vi "Save_Position_Checking.vi"(2 "Traverse Name":string, 3 "Error String":string, 4 "Model       Roll      Pitch       Yaw (deg)":sgl[](array[numeric]) format="%#.2f", 5 "Position":sgl[](array[numeric])=[0.0, 200.0, 40.0] format="%.2f") -> ()   [LabVIEW 2018]
uses:
  Collision_Detection/Triangles/EnFlo specific/Collision Detection global.vi
  Globals/Constants_global.vi
  Globals/Trav_pos_global.vi
panel:
  out "appended array":string[](array[string])
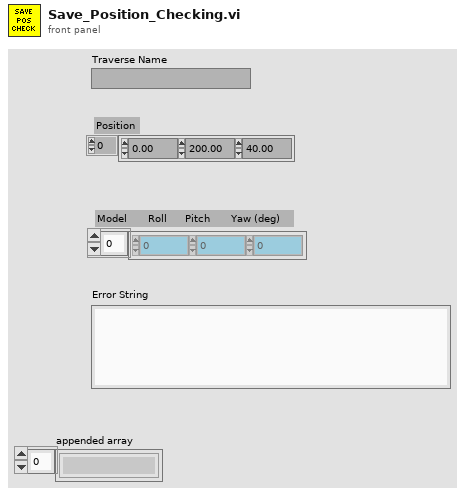
[diagram p1: front panel]
types:
  T1 = typedef "Traverse_cluster.ctl" = cluster{"Start X":sgl, "Start Y":sgl, "Start Z":sgl, "End X":sgl, "End Y":sgl, "End Z":sgl, "No. of pts.":i32, "Spacing":T2, "Filename":path, "Tunnel Speed":dbl, "Averaging time (min)":dbl, "Extra Commands":string, "Carrier_1 Q (l/min)":dbl, "Carrier_2 Q (l/min)":dbl, "Trace Gas Concentration (%)":dbl, "Specific Arguments":string, "Comments":string, "Row No":i32, "Row Type Selector":T3, "Completion time":string, "Row Duration (mins)":dbl, "No. of Valid pts.":i32, "Meas Setup File":string}
  T2 = typedef "Spacing.ctl" = enum16{"Linear", "Log", "Gauss", "Specified", "N/A"}
  T3 = typedef "Multi_run_mode.ctl" = enum16{"Move Traverse Only", "Set Tunnel Speed Only", "Set Source Only", "Set Measurement Conditions", "Single Measurement", "Vertical Profile", "Lateral Profile", "Longitudinal Profile", "Multi-Axis Profile", "Explore Volume", "Auto Calibrate", "Meas Fast FID Bkgnd", "Check Beam Power", "Scanning Valve Measurement", "Run VI Named:", "Set ADAM Ch", "Wait (minutes)", "Send Message", "Synchronize With:", "Fall Back to this Row", "Turn Off Row Repeating", "Traverse 3D Volume", "Blank Row", "Jump to Fall Back Row"}
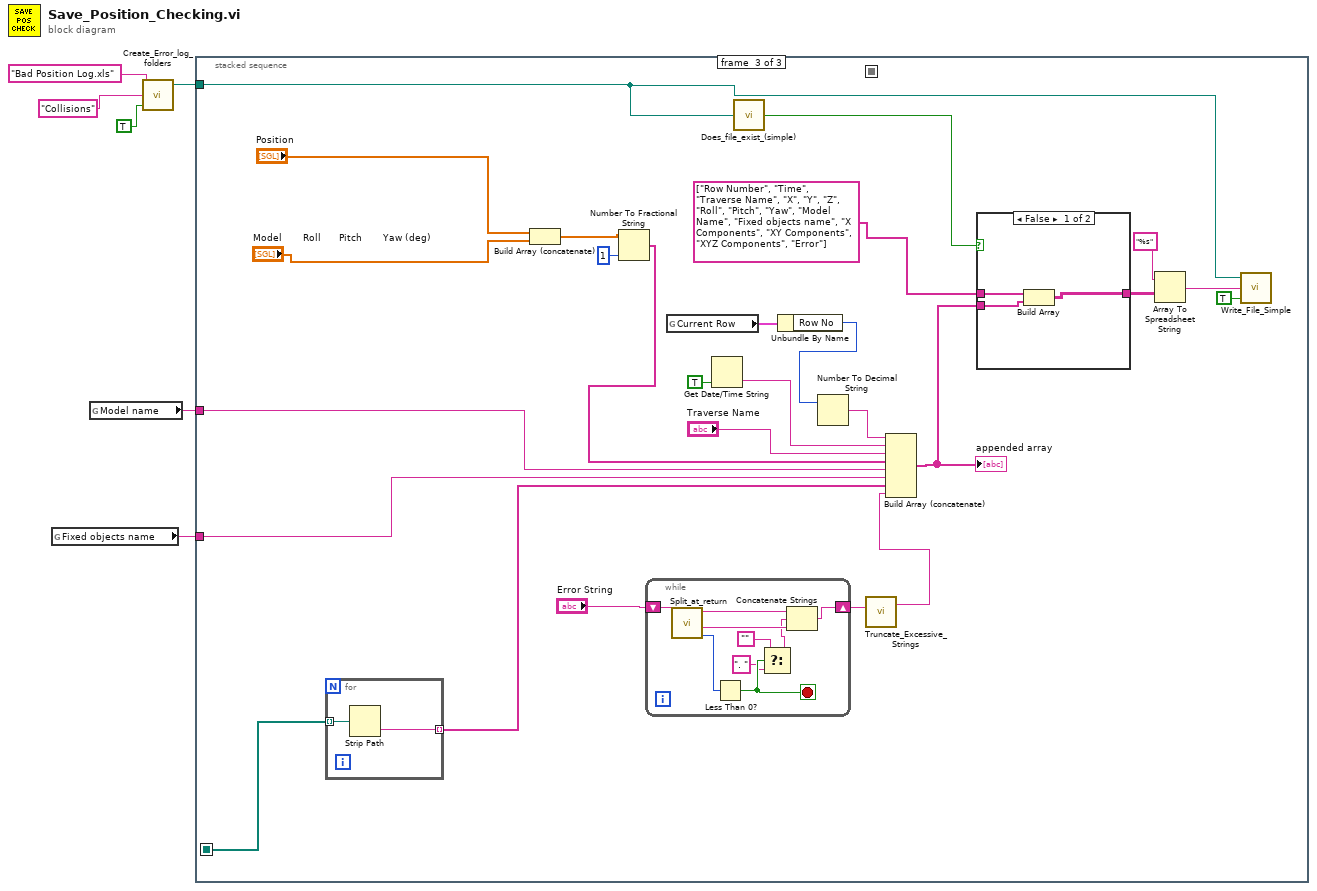
[diagram p0: block diagram]
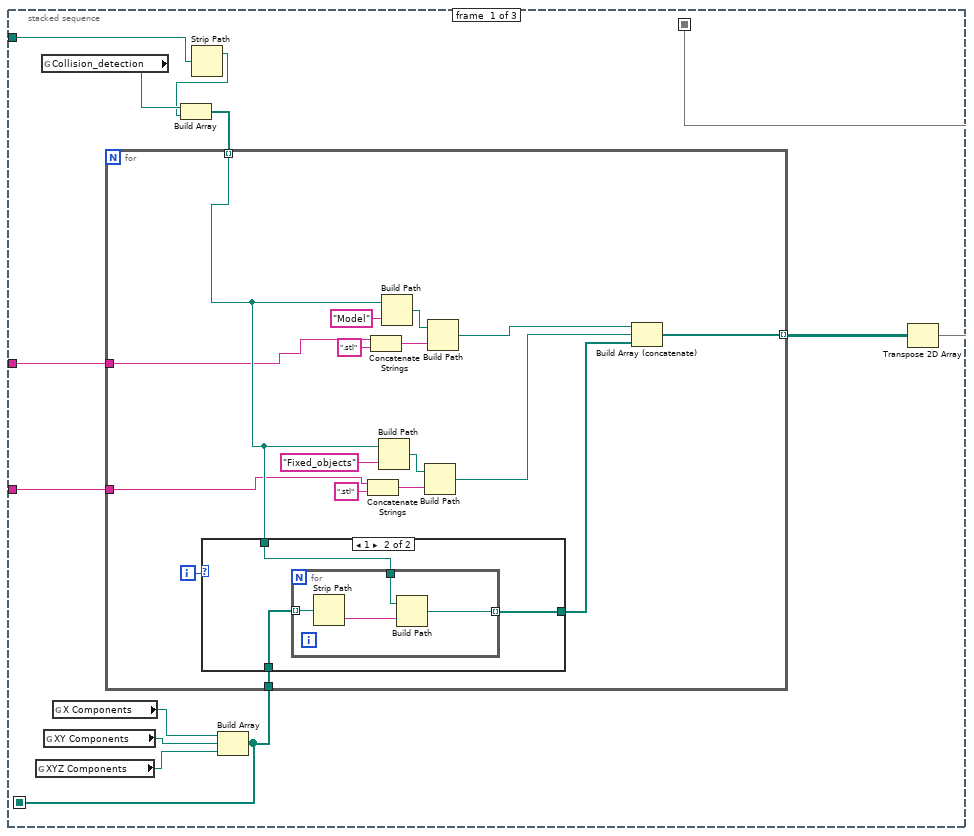
[diagram p2: hidden frame]
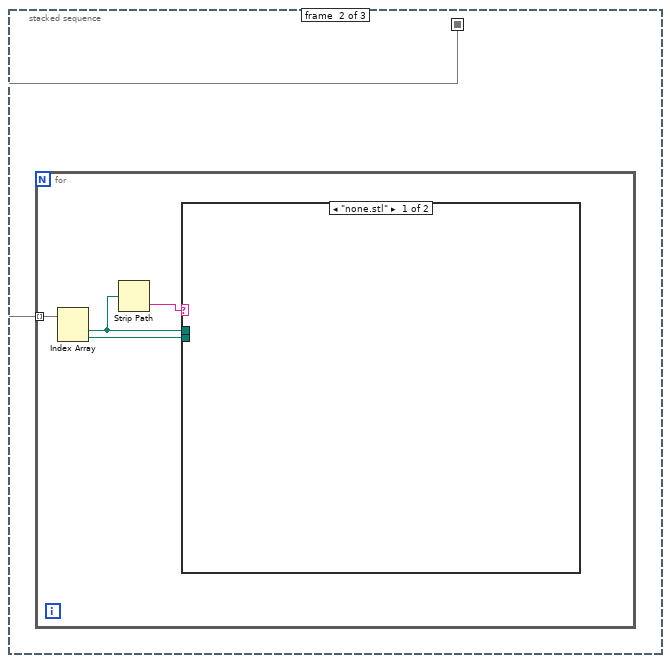
[diagram p4: hidden frame]
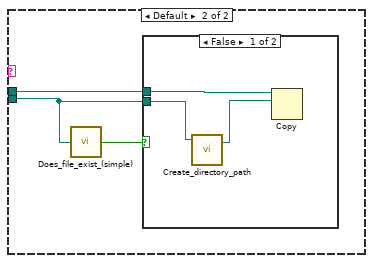
[diagram p5: hidden frame]
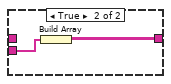
[diagram p7: hidden frame]
diagram:
  n1 = global read "Collision Detection global.vi" "Fixed objects name"() -> (w2:string)
  n2 = global read "Collision Detection global.vi" "Model name"() -> (w3:string)
  n3 = call "Create_Error_log_folders.vi"("Log Filename"="Bad Position Log.xls", "Log Folder"="Collisions", "Per Day Log File?"=TRUE) -> ("Local Log File"=w4:path)  [unwired: 3 in, 1 out]
  n4 = stacked-sequence {
    seq-local: [w14 _ _] -> [_ w44 _]
    seq-local: [w7 _ _] -> [_ _ w80]
    tunnel: w4 -> [w13 _ w62]
    tunnel: w3 -> [w12 _ w79]
    tunnel: w2 -> [w11 _ w78]
    frame #0 {
      n5 = global read "Collision Detection global.vi" "XYZ Components"() -> (w10:path)
      n6 = global read "Constants_global.vi" "Collision_detection"() -> (w18:path)
      n7 = global read "Collision Detection global.vi" "XY Components"() -> (w9:path)
      n8 = global read "Collision Detection global.vi" "X Components"() -> (w8:path)
      n9 = Strip Path(path=w13) -> (stripped path=w17:path)  [unwired: 1 out]
      n10 = Build Array(w18, w17) -> (w16:path[])
      n11 = Build Array(w8, w9, w10) -> (w7:path[])
      n12 = for {
        tunnel: w16 -> [w21] mode=indexing
        tunnel: [w25] -> w15 mode=indexing
        tunnel: w7 -> [w22]
        tunnel: w12 -> [w20]
        tunnel: w11 -> [w19]
        i -> [w24]
        n13 = case shown="1" w24 {
          tunnel: [w36 w37] -> w23
          tunnel: w22 -> [w36 w39]
          tunnel: w21 -> [_ w38]
          frame 0, Default {
          }
          frame 1 {
            n14 = for {
              tunnel: w39 -> [w43] mode=indexing
              tunnel: w38 -> [w41]
              tunnel: [w40] -> w37 mode=indexing
              n15 = Strip Path(path=w43) -> (name=w42:string)  [unwired: 1 out]
              n16 = Build Path(base path=w41, name or relative path=w42) -> (appended path=w40:path)
            }
          }
        }
        n17 = Concatenate Strings(w19, ".stl" ("string")) -> (w28:string)
        n18 = Concatenate Strings(w20, ".stl" ("string")) -> (w35:string)
        n19 = Build Path(base path=w21, name or relative path="Fixed_objects") -> (appended path=w29:path)
        n20 = Build Path(base path=w21, name or relative path="Model") -> (appended path=w33:path)
        n21 = Build Path(base path=w29, name or relative path=w28) -> (appended path=w26:path)
        n22 = Build Path(base path=w33, name or relative path=w35) -> (appended path=w27:path)
        n23 = Build Array (concatenate)(w27, w26, w23) -> (w25:path[])
      }
      n24 = Transpose 2D Array(2D array=w15) -> (transposed array=w14:path[][])
    }
    frame #1 {
      n25 = for {
        tunnel: w44 -> [w48] mode=indexing
        n26 = Index Array(array=w48) -> (element #1=w46:path, element #2=w47:path)  [unwired: 2 in]
        n27 = Strip Path(path=w46) -> (name=w45:string)  [unwired: 1 out]
        n28 = case shown="\"none.stl\"" w45 {
          tunnel: w47 -> [_ w50]
          tunnel: w46 -> [_ w49]
          frame "none.stl" {
          }
          frame Default {
            n29 = call "Does_file_exist_(simple).vi"("Pathname"=w50) -> ("exists?"=w51:bool)
            n30 = case shown="False" w51 {
              tunnel: w49 -> [w54 _]
              tunnel: w50 -> [w53 _]
              frame False {
                n31 = call "Create_directory_path.vi"("Path name"=w53) -> ("Path name Out"=w52:path)  [unwired: 2 in, 1 out]
                n32 = Copy(10:w52, 11:w54) -> ()  [unwired: 3 in, 3 out]
              }
              frame True {
              }
            }
          }
        }
      }
    }
    frame #2 {
      n33 = for {
        tunnel: w80 -> [w96] mode=indexing
        tunnel: [w95] -> w77 mode=indexing
        n34 = Strip Path(path=w96) -> (name=w95:string)  [unwired: 1 out]
      }
      n35 = Build Array (concatenate)("Position", "Model       Roll      Pitch       Yaw (deg)") -> (w74:sgl[])
      n36 = Number To Fractional String(number=w74, precision (6)=i16 1) -> (F-format string=w72:string[])  [unwired: 2 in]
      n37 = while {
        shift-right: [w92] -> w56
        shift-left: "Error String" -> [w94]
        stop <- w89 stop-if-true
        n38 = call "Split_at_return.vi"("String"=w94) -> ("before substring"=w93:string, "after substring"=w90:string, "offset past match"=w91:i32)  [unwired: 1 in, 1 out]
        n39 = Less Than 0?(x=w91) -> (x < 0?=w89:bool)
        n40 = Select(t="", s=w89, f=". " ("string")) -> (s? t:f=w86:string)
        n41 = Concatenate Strings(w93, w86, w90) -> (w92:string)
      }
      n42 = global read "Trav_pos_global.vi" "Current Row"() -> (w59:T1)
      n43 = Get Date/Time String(want seconds? (F)=TRUE) -> (time string=w70:string)  [unwired: 2 in, 1 out]
      n44 = call "Does_file_exist_(simple).vi"("Pathname"=w62) -> ("exists?"=w67:bool)
      n45 = Unbundle By Name(w59) -> ("Row No"=w58:i32)
      n46 = Number To Decimal String(number=w58) -> (decimal integer string=w57:string)  [unwired: 1 in]
      n47 = call "Truncate_Excessive_Strings.vi"("String"=w56) -> ("Truncated String"=w55:string)  [unwired: 2 in]
      n48 = Build Array (concatenate)(w57, w70, "Traverse Name", w72, w79, w78, w77, w55) -> (w66:string[])
      "appended array" <- w66
      n49 = case shown="False" w67 {
        tunnel: w66 -> [w83 w85]
        tunnel: [w81 w84] -> w65
        tunnel: string[] ["Row Number", "Time", "Traverse Name", "X", "Y", "Z", "Roll", "Pitch", "Yaw", "Model Name", "Fixed objects name", "X Components", "XY Components", "XYZ Components", "Error"] ("appended array") -> [w82 _]
        frame False {
          n50 = Build Array(w82, w83) -> (w81:string[][])
        }
        frame True {
          n51 = Build Array(w85) -> (w84:string[][])
        }
      }
      n52 = Array To Spreadsheet String(array=w65, 3:"%s" ("format string")) -> (spreadsheet string=w61:string)  [unwired: 1 in]
      n53 = call "Write_File_Simple.vi"("append to file? (new file:F)"=TRUE, "character string"=w61, "file path"=w62) -> ()  [unwired: 2 out]
    }
  }
